vi "Emballage scan produit a emballer_FLAT.vi"(5 "error in (no error)":errorcluster caption="entrée d'erreur (pas d'erreur)") -> (0 "error out":errorcluster caption="sortie d'erreur", 1 "Nom du produit":string, 2 "Paramètres Produit (PP)":T1={"Numéro T121"="F120023", "Créateur"="LGU", "Date de création"="15/02/2008", "Date de modification"="15/02/2008", "indice produit"="", "Code Barre fixe"="12216C0125", "Affiche n° Client [Oui/Non]"="oui", "Fichier PTV"="Famille_PTV", "Nbr de valves / Cartons"="50", "Mélange des lots posiible [Oui/Non] "="expedition@fas.ch", "Affiche code barre client [Oui/Non]"="", "Fichier PP valve sur embase"="", "Valve Direct/Compensée [D/C]"="D"}, 3 "Arrêter le programme (T)":bool)   [LabVIEW 2020]
uses:
  Flatprop/Flatprop - Standard/XML/Control/PP Param_3.ctl
  Modules/FS/60_FS_Controles/60_FS_SetGet.ctl
panel:
  out "Résultat scanner":string
  in  "liste":bool
  in  "Scanner":bool
  out "Scanner ou liste":string="Voulez-vous scanner la pièce ou la choisir sur la liste ?"
  in  "Bouton OK":bool
  in  "Annuler?":bool
  # "Choix du produit à emballer"
  # "etiquette"
  # "(Lien interchangeable)"
  # "emballage"
  # "emballage"
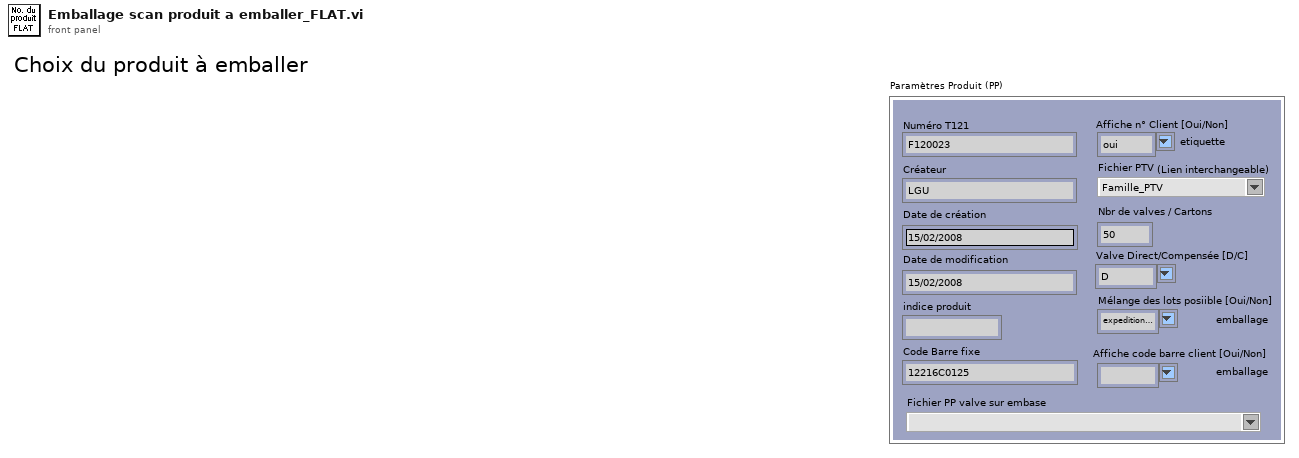
[diagram p1: front panel]
types:
  T1 = typedef "PP Param_3.ctl" = cluster{"Numéro T121":string, "Créateur":string, "Date de création":string, "Date de modification":string, "indice produit":string, "Code Barre fixe":string, "Affiche n° Client [Oui/Non]":string, "Fichier PTV":string, "Nbr de valves / Cartons":string, "Mélange des lots posiible [Oui/Non] ":string, "Affiche code barre client [Oui/Non]":string, "Fichier PP valve sur embase":string, "Valve Direct/Compensée [D/C]":string}
  T2 = typedef "60_FS_SetGet.ctl" = enum16{"set", "get"}
  T3 = cluster{"Admin-réseau":path, "XML-Réseau":path, " Résultat tests-Réseau":path, " Archive prôbleme-Réseau":path, " Archive Test  Local":path}
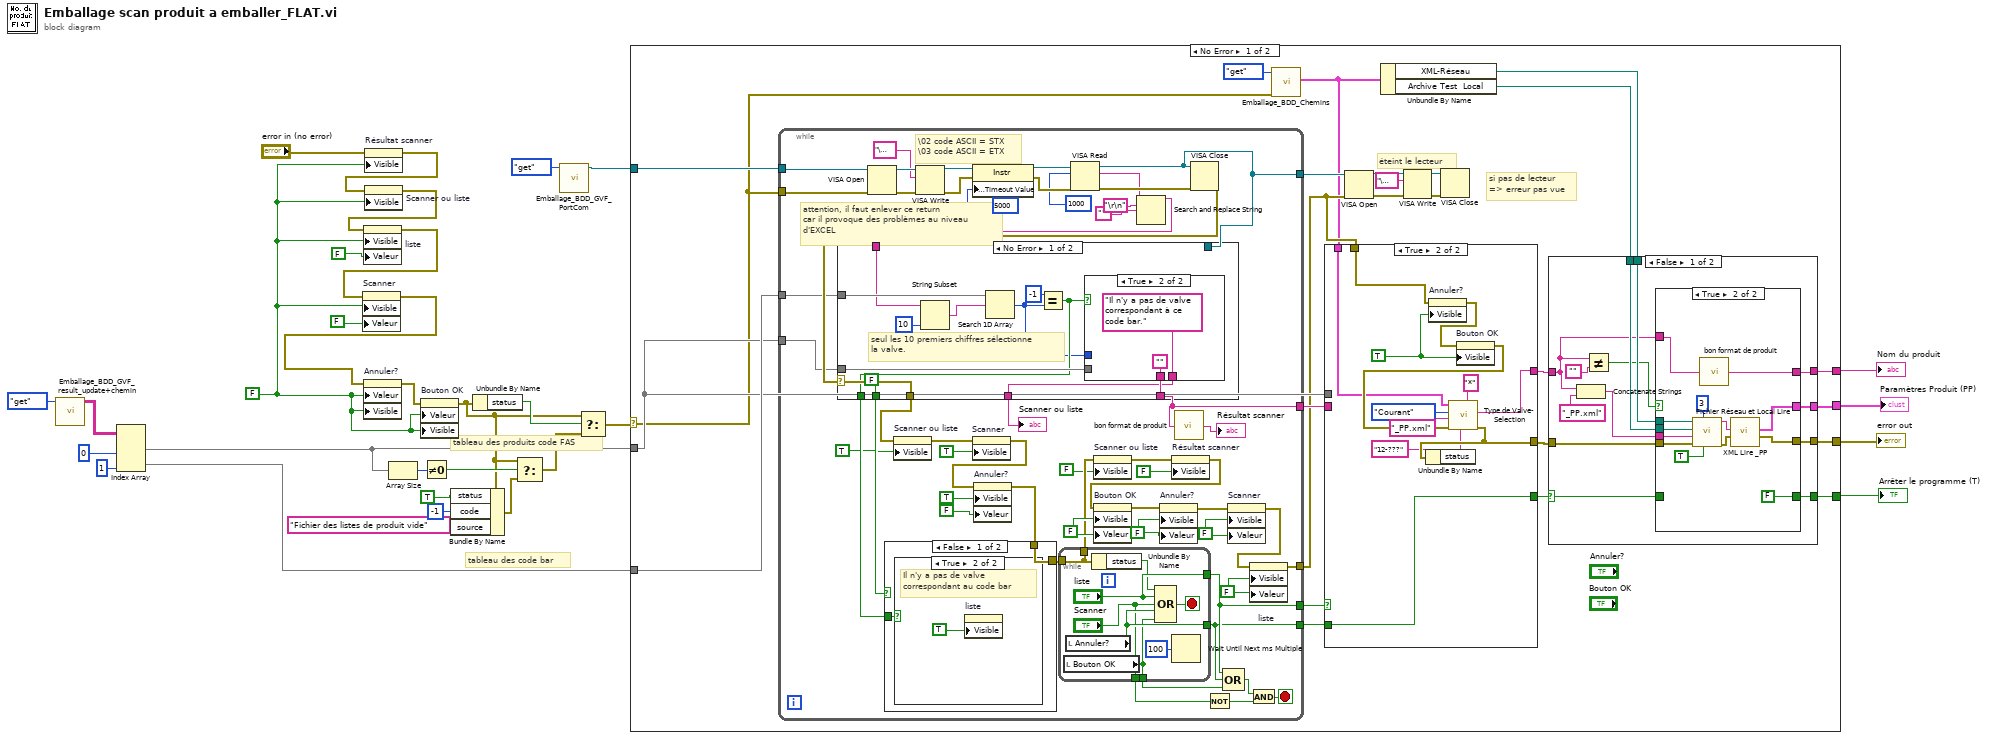
[diagram p0: block diagram]
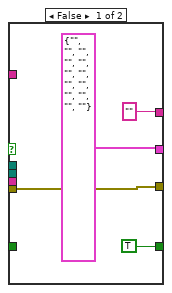
[diagram p2: hidden frame]
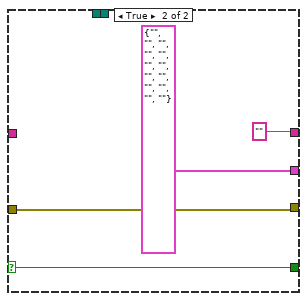
[diagram p3: hidden frame]
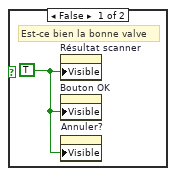
[diagram p4: hidden frame]
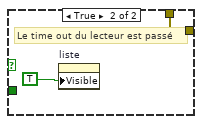
[diagram p5: hidden frame]
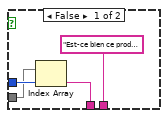
[diagram p6: hidden frame]
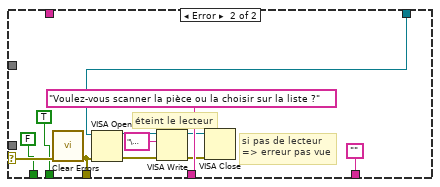
[diagram p7: hidden frame]
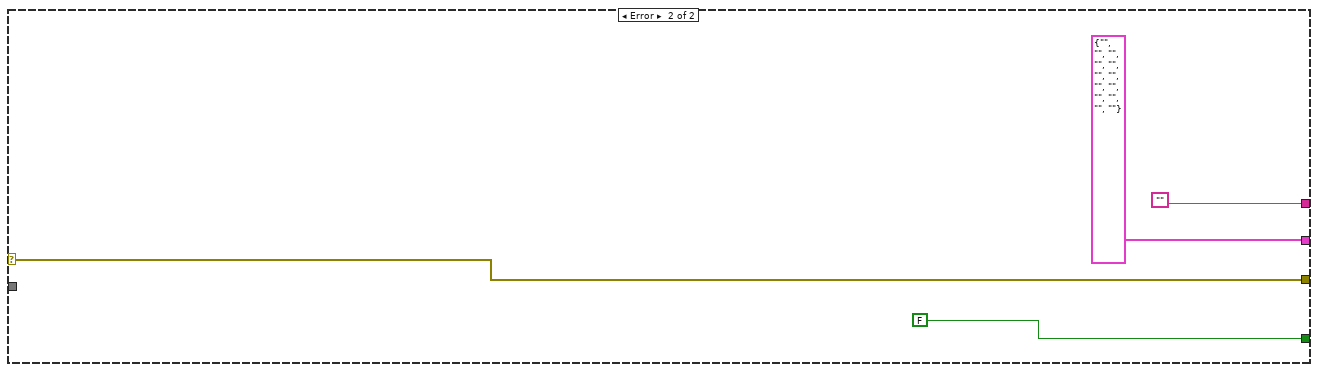
[diagram p9: hidden frame]
diagram:
  w14 = FALSE
  # "tableau des produits code FAS"
  # "tableau des code bar"
  n1 = call "Emballage_BDD_GVF_result_update+chemin.vi"("Énum"=enum16{"get", "set"}."get") -> ("Tab codif-code bar OUT"=w4:string[][])  [unwired: 9 in, 1 out]
  n2 = Index Array(array=w4, index (col) #1=0 ("indice désactivé (col)"), index (col) #2=1 ("indice (col)")) -> (element #1=w5:string[], element #2=w6:string[])  [unwired: 2 in]
  n3 = property on="Résultat scanner" class="Str"(error in="error in (no error)", "Visible"=w14) -> (error out=w16:errorcluster)  [unwired: 1 in, 1 out]
  n4 = property on="Scanner ou liste" class="Str"(error in=w16, "Visible"=w14) -> (error out=w15:errorcluster)  [unwired: 1 in, 1 out]
  n5 = property on="liste" class="Bool (strict)"(error in=w15, "Visible"=w14, "Valeur"=FALSE) -> (error out=w9:errorcluster)  [unwired: 1 in, 1 out]
  n6 = property on="Scanner" class="Bool (strict)"(error in=w9, "Visible"=w14, "Valeur"=FALSE) -> (error out=w11:errorcluster)  [unwired: 1 in, 1 out]
  n7 = property on="Annuler?" class="Bool (strict)"(error in=w11, "Valeur"=w14, "Visible"=w14) -> (error out=w30:errorcluster)  [unwired: 1 in, 1 out]
  n8 = Array Size(array=w5) -> (size(s)=w27:i32)
  n9 = property on="Bouton OK" class="Bool (strict)"(error in=w30, "Valeur"=w14, "Visible"=w14) -> (error out=w18:errorcluster)  [unwired: 1 in, 1 out]
  n10 = Not Equal To 0?(x=w27) -> (x != 0?=w21:bool)
  n11 = Bundle By Name(cluster=w18, "status"=TRUE, "code"=-1, "source"="Fichier des listes de produit vide") -> (w20:errorcluster)
  n12 = Unbundle By Name(w18) -> ("status"=w23:bool)
  n13 = Select(t=w18, s=w21, f=w20) -> (s? t:f=w19:errorcluster)
  n14 = call "Emballage_BDD_GVF_PortCom.vi"("Énum"=enum16{"get", "set"}."get") -> ("PortCom Scanner"=w2:refnum<visa-resource-name>)  [unwired: 8 in, 2 out]
  n15 = Select(t=w18, s=w23, f=w19) -> (s? t:f=w22:errorcluster)
  n16 = case shown="No Error" w22 {
    selector: w22 -> [w32 w207]
    tunnel: [w44 w207] -> w31
    tunnel: w5 -> [w45 _]
    tunnel: [w37 FALSE] -> w28
    tunnel: [w40 ""] -> w29
    tunnel: w2 -> [w50 _]
    tunnel: w6 -> [w49 _]
    tunnel: [w42 T1 {"Numéro T121"="", "Créateur"="", "Date de création"="", "Date de modification"="", "indice produit"="", "Code Barre fixe"="", "Affiche n° Client [Oui/Non]"="", "Fichier PTV"="", "Nbr de valves / Cartons"="", "Mélange des lots posiible [Oui/Non] "="", "Affiche code barre client [Oui/Non]"="", "Fichier PP valve sur embase"="", "Valve Direct/Compensée [D/C]"=""} ("Paramètres Produit (PP)")] -> w10
    frame No Error {
      # "si pas de lecteur\n=> erreur pas vue"
      # "éteint le lecteur"
      n17 = while {
        tunnel: w50 -> [w136]
        tunnel: w32 -> [w135]
        tunnel: [w113] -> w51
        tunnel: [w108] -> w38
        tunnel: [w95] -> w47
        tunnel: w49 -> [w128]
        tunnel: w45 -> [w127]
        tunnel: [w112] -> w48
        tunnel: [w92] -> w46
        stop <- w117 stop-if-true
        w104 = FALSE
        w105 = FALSE
        w106 = FALSE
        w107 = FALSE
        # "attention, il faut enlever ce return\ncar il provoque des problèmes au niveau\nd'EXCEL"
        # "\\02 code ASCII = STX\n\\03 code ASCII = ETX"
        n18 = VISA Open(error in (no error)=w135, VISA resource name=w136) -> (VISA resource name=w143:refnum<visa-resource-name>, error out=w144:errorcluster)  [unwired: 3 in]
        n19 = VISA Write(VISA resource name=w143, write buffer="\u0002", error in (no error)=w144) -> (VISA resource name out=w141:refnum<visa-resource-name>, error out=w142:errorcluster)  [unwired: 1 out]
        n20 = property class="Instr"(reference=w141, error in=w142, "General Settings:Timeout Value"=u32 5000 ("Tmo Value")) -> (reference out=w139:refnum<visa-resource-name>, error out=w140:errorcluster)
        n21 = VISA Read(VISA resource name=w139, byte count=u32 1000 ("byte count (0)"), error in (no error)=w140) -> (VISA resource name out=w95:refnum<visa-resource-name>, read buffer=w132:string, error out=w134:errorcluster)  [unwired: 1 out]
        n22 = Search and Replace String(input string=w132, search string="\r\n", replace string="") -> (result string=w93:string)  [unwired: 5 in, 3 out]
        n23 = VISA Close(VISA resource name=w95, error in (no error)=w134) -> (error out=w133:errorcluster)
        n24 = case shown="No Error" w133 {
          selector: w133 -> [w170 w188]
          tunnel: [w170 w177] -> w123
          tunnel: [w166 "Voulez-vous scanner la pièce ou la choisir sur la liste ?"] -> w125
          tunnel: w128 -> [w163 _]
          tunnel: w93 -> [w161 _]
          tunnel: w127 -> [w169 _]
          tunnel: [w165 FALSE] -> w126
          tunnel: [FALSE TRUE] -> w124
          tunnel: [w167 ""] -> w92
          tunnel: w95 -> [_ w178]
          frame No Error {
            # "seul les 10 premiers chiffres sélectionne\nla valve."
            n25 = String Subset(string=w161, length (rest)=10 ("longueur (reste)")) -> (substring=w160:string)  [unwired: 1 in]
            n26 = Search 1D Array(1D array=w163, element=w160) -> (index of element=w162:i32)  [unwired: 1 in]
            n27 = Equal?(x=-1, y=w162) -> (x = y?=w165:bool)
            n28 = case shown="True" w165 {
              tunnel: w162 -> [w173 _]
              tunnel: w169 -> [w171 _]
              tunnel: ["Est-ce bien ce produit que vous voulez tester ?" "Il n'y a pas de valve correspondant à ce code bar."] -> w166
              tunnel: [w172 ""] -> w167
              frame False {
                n29 = Index Array(array=w171, index=w173) -> (element=w172:string)
              }
              frame True {
              }
            }
          }
          frame Error {
            # "si pas de lecteur\n=> erreur pas vue"
            # "éteint le lecteur"
            n30 = call <vilib>:"Clear Errors.vi"("error in (no error)"=w188) -> ("error out"=w177:errorcluster)  [unwired: 5 in, 1 out]
            n31 = VISA Open(error in (no error)=w177, VISA resource name=w178) -> (VISA resource name=w180:refnum<visa-resource-name>, error out=w182:errorcluster)  [unwired: 3 in]
            n32 = VISA Write(VISA resource name=w180, write buffer="\u0003", error in (no error)=w182) -> (VISA resource name out=w179:refnum<visa-resource-name>, error out=w181:errorcluster)  [unwired: 1 out]
            n33 = VISA Close(VISA resource name=w179, error in (no error)=w181) -> ()  [unwired: 1 out]
          }
        }
        "Scanner ou liste" <- w125
        n34 = property on="Scanner ou liste" class="Str"(error in=w123, "Visible"=TRUE) -> (error out=w121:errorcluster)  [unwired: 1 in, 1 out]
        n35 = property on="Scanner" class="Bool (strict)"(error in=w121, "Visible"=TRUE) -> (error out=w97:errorcluster)  [unwired: 1 in, 1 out]
        n36 = property on="Annuler?" class="Bool (strict)"(error in=w97, "Visible"=TRUE, "Valeur"=FALSE) -> (error out=w96:errorcluster)  [unwired: 1 in, 1 out]
        n37 = case shown="False" w124 {
          tunnel: w96 -> [w154 w158]
          tunnel: [w154 w158] -> w119
          tunnel: w126 -> [w153 _]
          frame False {
            n38 = case shown="True" w153 {
              frame False {
                w155 = TRUE
                # "Est-ce bien la bonne valve"
                n39 = property on="Résultat scanner" class="Str"("Visible"=w155) -> ()  [unwired: 2 in, 2 out]
                n40 = property on="Bouton OK" class="Bool (strict)"("Visible"=w155) -> ()  [unwired: 2 in, 2 out]
                n41 = property on="Annuler?" class="Bool (strict)"("Visible"=w155) -> ()  [unwired: 2 in, 2 out]
              }
              frame True {
                # "Il n'y a pas de valve\ncorrespondant au code bar"
                n42 = property on="liste" class="Bool (strict)"("Visible"=TRUE) -> ()  [unwired: 2 in, 2 out]
              }
            }
          }
          frame True {
            # "Le time out du lecteur est passé"
            n43 = property on="liste" class="Bool (strict)"("Visible"=TRUE) -> ()  [unwired: 2 in, 2 out]
          }
        }
        n44 = while {
          tunnel: [w150] -> w112
          tunnel: ["liste"] -> w113
          tunnel: w119 -> [w146]
          tunnel: [w146] -> w103
          tunnel: [w148] -> w114
          tunnel: ["Scanner"] -> w115
          stop <- w152 stop-if-true
          n45 = local read "Bouton OK"() -> (w148:bool)
          n46 = local read "Annuler?"() -> (w150:bool)
          n47 = Unbundle By Name(w146) -> ("status"=w145:bool)
          n48 = Compound Arithmetic op=OR(w145, "liste", "Scanner", w150, w148) -> (w152:bool)
          n49 = Wait Until Next ms Multiple(millisecond multiple=100) -> ()  [unwired: 1 out]
        }
        n50 = property on="Scanner ou liste" class="Str"(error in=w103, "Visible"=FALSE) -> (error out=w102:errorcluster)  [unwired: 1 in, 1 out]
        n51 = property on="Résultat scanner" class="Str"(error in=w102, "Visible"=FALSE) -> (error out=w101:errorcluster)  [unwired: 1 in, 1 out]
        n52 = property on="Bouton OK" class="Bool (strict)"(error in=w101, "Visible"=w104, "Valeur"=w104) -> (error out=w111:errorcluster)  [unwired: 1 in, 1 out]
        n53 = property on="Annuler?" class="Bool (strict)"(error in=w111, "Visible"=w105, "Valeur"=w105) -> (error out=w110:errorcluster)  [unwired: 1 in, 1 out]
        n54 = call "bon format de produit.vi"("Chaîne"=w92) -> ("Chaîne 2"=→"Résultat scanner":string)
        n55 = Not(x=w115) -> (.not. x?=w116:bool)
        n56 = Compound Arithmetic op=OR(w113, w112, w114) -> (w118:bool)
        n57 = property on="Scanner" class="Bool (strict)"(error in=w110, "Visible"=w106, "Valeur"=w106) -> (error out=w109:errorcluster)  [unwired: 1 in, 1 out]
        n58 = property on="liste" class="Bool (strict)"(error in=w109, "Visible"=w107, "Valeur"=w107) -> (error out=w108:errorcluster)  [unwired: 1 in, 1 out]
        n59 = And(x=w118, y=w116) -> (x .and. y?=w117:bool)
      }
      n60 = call "Emballage_BDD_Chemins.vi"("error in (no error)"=w32, "SetGet"=60_FS_SetGet."get") -> ("CLT_Chemins_out"=w34:T3)  [unwired: 8 in, 1 out]
      n61 = case shown="True" w51 {
        tunnel: [w190 w203] -> w43
        tunnel: w45 -> [_ _]
        tunnel: [w191 w194] -> w39
        tunnel: w48 -> [w191 w194]
        tunnel: w38 -> [w190 w198]
        tunnel: w46 -> [w189 _]
        tunnel: w34 -> [_ w199]
        tunnel: [w189 w197] -> w41
        frame False {
        }
        frame True {
          w202 = TRUE
          n62 = property on="Annuler?" class="Bool (strict)"(error in=w198, "Visible"=w202) -> (error out=w200:errorcluster)  [unwired: 1 in, 1 out]
          n63 = property on="Bouton OK" class="Bool (strict)"(error in=w200, "Visible"=w202) -> (error out=w201:errorcluster)  [unwired: 1 in, 1 out]
          n64 = call "Type de Valve- Selection.vi"("Flitre raccord"="*", "Flitre article"="12-???", "error in"=w201, "Extension fin"="_PP.xml", "Dernier filtre"=enum16{"Tension", "Courant"}."Courant", "Chemins"=w199) -> ("error out"=w203:errorcluster, "Nom de la config"=w197:string)  [unwired: 3 in]
          n65 = Unbundle By Name(w203) -> ()  [unwired: 1 out]
        }
      }
      n66 = VISA Open(error in (no error)=w38, VISA resource name=w47) -> (VISA resource name=w53:refnum<visa-resource-name>, error out=w55:errorcluster)  [unwired: 3 in]
      n67 = Unbundle By Name(w34) -> ("XML-Réseau"=w36:path, "Archive Test  Local"=w35:path)
      n68 = VISA Write(VISA resource name=w53, write buffer="\u0003", error in (no error)=w55) -> (VISA resource name out=w52:refnum<visa-resource-name>, error out=w54:errorcluster)  [unwired: 1 out]
      n69 = VISA Close(VISA resource name=w52, error in (no error)=w54) -> ()  [unwired: 1 out]
      n70 = case shown="False" w39 {
        selector: w39 -> [w59 w87]
        tunnel: [w63 w90] -> w44
        tunnel: w43 -> [w69 w90]
        tunnel: w36 -> [w68 _]
        tunnel: w35 -> [w67 _]
        tunnel: [w62 T1 {"Numéro T121"="", "Créateur"="", "Date de création"="", "Date de modification"="", "indice produit"="", "Code Barre fixe"="", "Affiche n° Client [Oui/Non]"="", "Fichier PTV"="", "Nbr de valves / Cartons"="", "Mélange des lots posiible [Oui/Non] "="", "Affiche code barre client [Oui/Non]"="", "Fichier PP valve sur embase"="", "Valve Direct/Compensée [D/C]"=""} ("Paramètres Produit (PP)")] -> w42
        tunnel: w41 -> [w57 _]
        tunnel: [w64 "" ("Chaîne 2")] -> w40
        tunnel: [w58 w87] -> w37
        frame False {
          n71 = Concatenate Strings(w57, "_PP.xml" ("Extension fin")) -> (w65:string)
          n72 = Not Equal?(x=w57, y="") -> (x != y?=w60:bool)
          n73 = case shown="True" w60 {
            tunnel: w69 -> [w71 w86]
            tunnel: w68 -> [_ w84]
            tunnel: w67 -> [_ w83]
            tunnel: w65 -> [_ w82]
            tunnel: ["" ("Chaîne 2") w80] -> w64
            tunnel: [w71 w78] -> w63
            tunnel: [T1 {"Numéro T121"="", "Créateur"="", "Date de création"="", "Date de modification"="", "indice produit"="", "Code Barre fixe"="", "Affiche n° Client [Oui/Non]"="", "Fichier PTV"="", "Nbr de valves / Cartons"="", "Mélange des lots posiible [Oui/Non] "="", "Affiche code barre client [Oui/Non]"="", "Fichier PP valve sur embase"="", "Valve Direct/Compensée [D/C]"=""} ("Paramètres Produit (PP)") w76] -> w62
            tunnel: w59 -> [_ _]
            tunnel: [TRUE FALSE] -> w58
            tunnel: w57 -> [_ w74]
            frame False {
            }
            frame True {
              n74 = call "Fichier Réseau et Local Lire .vi"("reseau prioritaire ?"=TRUE, "nbr de sous dossier"=3, "error in"=w86, "Nom fichier"=w82, "Dossier Local"=w83, "Fichier ou dossier Reseau"=w84) -> ("error out"=w79:errorcluster, "Texte"=w77:string)  [unwired: 1 in, 2 out]
              n75 = call "bon format de produit.vi"("Chaîne"=w74) -> ("Chaîne 2"=w80:string)
              n76 = call "XML Lire _PP.vi"("XML _PP"=w77, "error in"=w79) -> ("Paramètres Produit"=w76:T1, "error out"=w78:errorcluster)  [unwired: 7 in]
            }
          }
        }
        frame True {
        }
      }
    }
    frame Error {
    }
  }
  "error out" <- w31
  "Arrêter le programme (T)" <- w28
  "Nom du produit" <- w29
  "Paramètres Produit (PP)" <- w10
